vi "niRFUtil TRC Waveform to Trace (real WDT).vi"(7 "Real WDT":T1) -> (8 "Measurement Trace":T2 format="%.2f")   [LabVIEW 2015, in "niRFUtil.lvlib"]
doc: "(c) Copyright 2006, National Instruments, Inc. This VI may not be duplicated, sold, or distributed without written consent from National Instruments."
uses:
  niRFUtil.lvlib
  Includes/niRFUtil INC Trace.ctl
  Includes/niRFUtil INC Real WDT.ctl
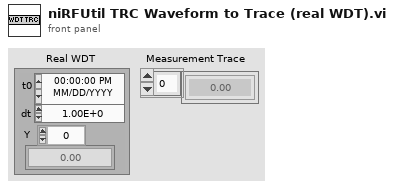
[diagram p1: front panel]
types:
  T1 = typedef "niRFUtil.lvlib/niRFUtil INC Real WDT.ctl" = waveform(sgl)
  T2 = typedef "niRFUtil.lvlib/niRFUtil INC Trace.ctl" = sgl[]
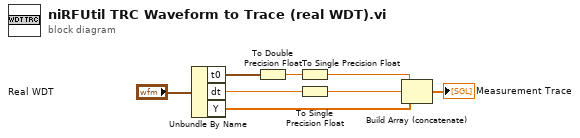
[diagram p0: block diagram]
diagram:
  n1 = Unbundle By Name("Real WDT") -> ("t0"=w6:timestamp, "dt"=w4:dbl, "Y"=w3:sgl[])
  n2 = To Double Precision Float(number=w6) -> (double precision float=w5:dbl)
  n3 = To Single Precision Float(number=w5) -> (single precision float=w2:sgl)
  n4 = To Single Precision Float(number=w4) -> (single precision float=w1:sgl)
  n5 = Build Array (concatenate)(w2, w1, w3) -> (→"Measurement Trace":sgl[])
